vi "Init Events.vi"(8 "error in (no error)":errorcluster, 11 "GWebAppArrayPanel in":refnum<class "GWebAppArrayPanel.lvclass">) -> (0 "error out":errorcluster, 3 "GWebAppArrayPanel out":refnum<class "GWebAppArrayPanel.lvclass">)   [LabVIEW 2020, in "PicoG-App.lvlib" / "GWebAppArrayPanel.lvclass"]
uses:
  GWebAppArrayPanel.lvclass
  GWebAppArrayPanel.lvclass/GWebAppArrayPanel.ctl
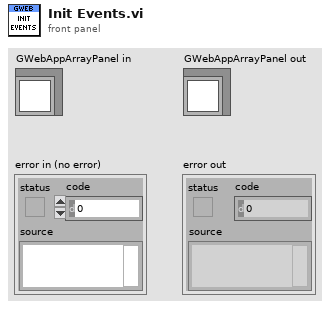
[diagram p1: front panel]
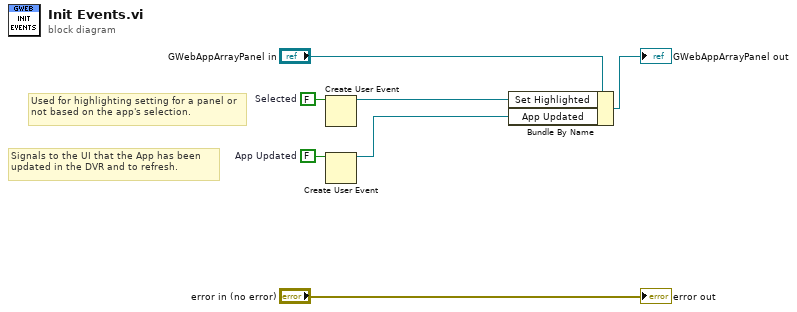
[diagram p0: block diagram]
diagram:
  w2 = FALSE  # App Updated
  w5 = FALSE  # Selected
  # "Signals to the UI that the App has been updated in the DVR and to refresh."
  # "Used for highlighting setting for a panel or not based on the app's selection."
  n1 = Create User Event(user event datatype=w5) -> (user event=w3:refnum<user-event>)  [unwired: 1 in, 1 out]
  n2 = Create User Event(user event datatype=w2) -> (user event=w1:refnum<user-event>)  [unwired: 1 in, 1 out]
  n3 = Bundle By Name(cluster="GWebAppArrayPanel in", "Set Highlighted"=w3, "App Updated"=w1) -> (→"GWebAppArrayPanel out":refnum<class "GWebAppArrayPanel.lvclass">)
  "error out" <- "error in (no error)"
